vi "clFileReader_setReaderPropertys.vi"(8 "blocklen (>=0) if you want to change this value":i32=-1, 9 "hiddenoffset (>=0) if you want to change this value":i32=-1, 10 "changeType":enum16{"changeValues", "ResetToFile"}(ring), 11 "clFileReader.lvclass IN":refnum<class "clFileReader.lvclass">) -> (3 "clFileReader.lvclass OUT":refnum<class "clFileReader.lvclass">)   [LabVIEW 2021, in "vi_lib.lvlib" / "clFileReader.lvclass"]
uses:
  clFileReader.lvclass
  clFileReader.lvclass/clFileReader.ctl
  clFile/clFile.lvclass
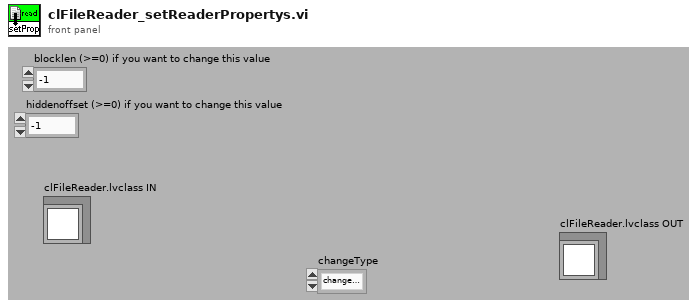
[diagram p1: front panel]
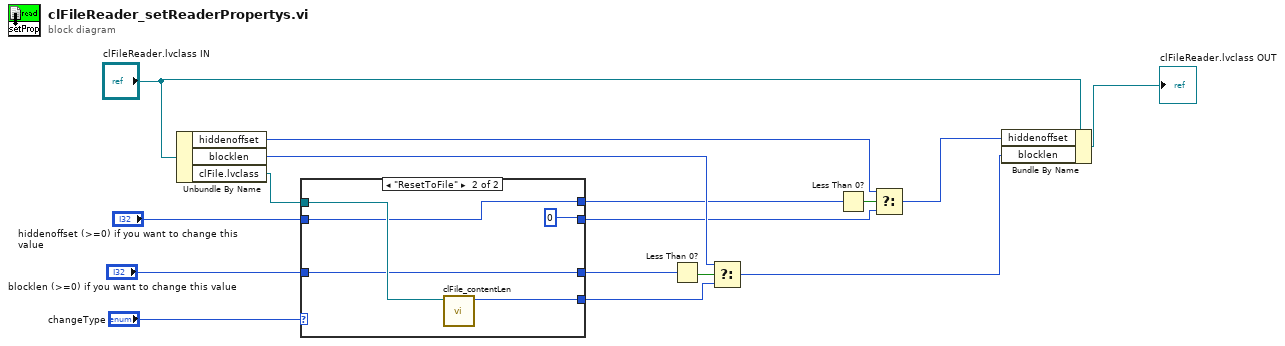
[diagram p0: block diagram]
diagram:
  n1 = Unbundle By Name("clFileReader.lvclass IN") -> ("hiddenoffset"=w12:u32, "blocklen"=w11:u32, "clFile.lvclass"=w7:refnum<class "clFile.lvclass">)
  n2 = case shown="\"ResetToFile\"" "changeType" {
    tunnel: w7 -> [_ w23]
    tunnel: "blocklen (>=0) if you want to change this value" -> [w18 w19]
    tunnel: [w18 w22] -> w5
    tunnel: [w17 0 ("hiddenoffset")] -> w3
    tunnel: "hiddenoffset (>=0) if you want to change this value" -> [w17 w20]
    tunnel: [w18 w19] -> w2
    tunnel: [w17 w20] -> w1
    frame "changeValues", Default {
    }
    frame "ResetToFile" {
      n3 = call "clFile_contentLen.vi"("clFile.lvclass"=w23) -> ("length"=w22:u32)  [unwired: 10 out]
    }
  }
  n4 = Less Than 0?(x=w2) -> (x < 0?=w10:bool)
  n5 = Select(t=w11, s=w10, f=w5) -> (s? t:f=w9:u32)
  n6 = Less Than 0?(x=w1) -> (x < 0?=w14:bool)
  n7 = Select(t=w12, s=w14, f=w3) -> (s? t:f=w13:u32)
  n8 = Bundle By Name(cluster="clFileReader.lvclass IN", "hiddenoffset"=w13, "blocklen"=w9) -> (→"clFileReader.lvclass OUT":refnum<class "clFileReader.lvclass">)
